vi "AMZ_S3_APIHLP_Parse HEAD Object Result.vi"(8 "error in (no error)":errorcluster, 11 "Response header":string) -> (0 "error out":errorcluster, 3 "HeadObjectResult":T1)   [LabVIEW 2015, in "LV Interface for Amazon S3.lvlib"]
uses:
  LV Interface for Amazon S3.lvlib
  Typedefs/AMZ_S3_API_HEADObjectResult.ctl
  Typedefs/AMZ_S3_API_GETObjectResult.ctl
  Typedefs/AMZ_S3_Key-Value pair.ctl
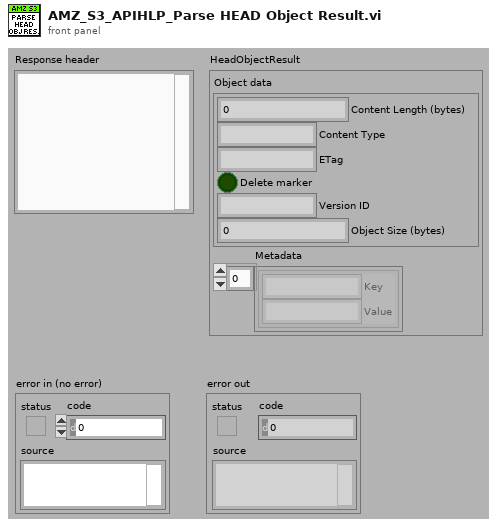
[diagram p1: front panel]
types:
  T1 = typedef "LV Interface for Amazon S3.lvlib/AMZ_S3_API_HEADObjectResult.ctl" = cluster{"Object data":T2, "Metadata":T3[]}
  T2 = typedef "LV Interface for Amazon S3.lvlib/AMZ_S3_API_GETObjectResult.ctl" = cluster{"Content Length (bytes)":u64, "Content Type":string, "ETag":string, "Delete marker":bool, "Version ID":string, "Object Size (bytes)":u64}
  T3 = typedef "LV Interface for Amazon S3.lvlib/AMZ_S3_Key-Value pair.ctl" = cluster{"Key":string, "Value":string}
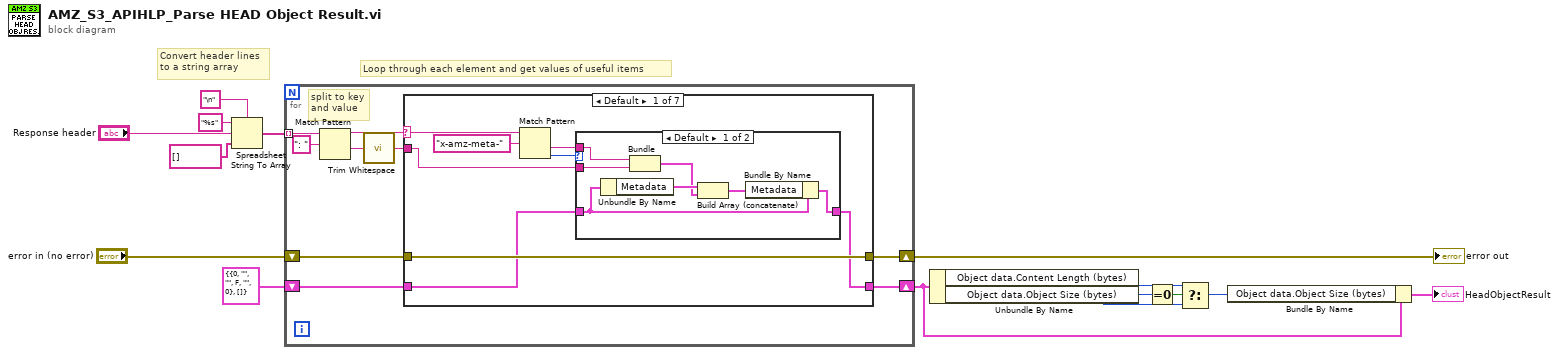
[diagram p0: block diagram]
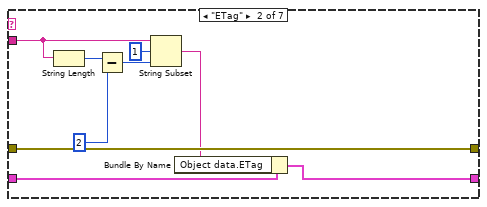
[diagram p3: hidden frame]
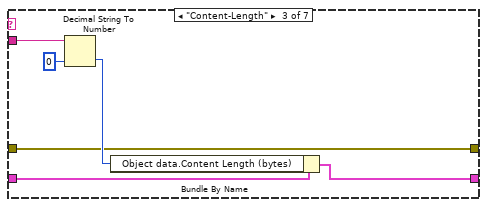
[diagram p4: hidden frame]
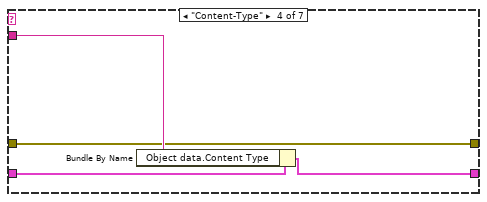
[diagram p5: hidden frame]
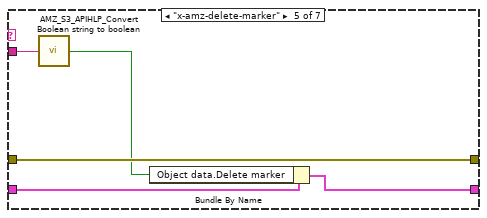
[diagram p6: hidden frame]
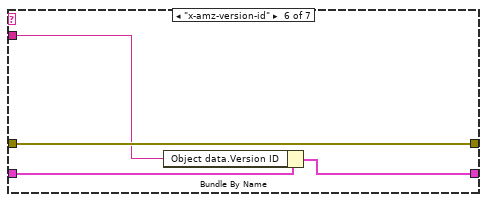
[diagram p7: hidden frame]
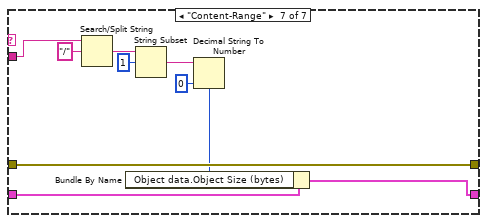
[diagram p8: hidden frame]
diagram:
  # "Loop through each element and get values of useful items"
  # "Convert header lines\nto a string array"
  n1 = Spreadsheet String To Array(delimiter (Tab)="\n", format string="%s", spreadsheet string="Response header", array type (2D Dbl)=string[] []) -> (array=w11:string[])
  n2 = for {
    tunnel: w11 -> [w23] mode=indexing
    shift-right: [w19] -> w7
    shift-left: "error in (no error)" -> [w20]
    shift-right: [w17] -> w3
    shift-left: T1 {"Object data"={"Content Length (bytes)"=0, "Content Type"="", "ETag"="", "Delete marker"=FALSE, "Version ID"="", "Object Size (bytes)"=0}, "Metadata"=[]} ("HeadObjectResult") -> [w18]
    # "split to key\nand value"
    n3 = Match Pattern(string=w23, regular expression=": ") -> (before substring=w21:string, after substring=w16:string)  [unwired: 1 in, 2 out]
    n4 = call <vilib>:"Trim Whitespace.vi"("string"=w16) -> ("trimmed string"=w15:string)  [unwired: 1 in]
    n5 = case shown="Default" w21 {
      selector: w21 -> [w30 _ _ _ _ _ _]
      tunnel: [w31 w48 w49 w55 w61 w65 w73] -> w19
      tunnel: w20 -> [w31 w48 w49 w55 w61 w65 w73]
      tunnel: w15 -> [w26 w46 w54 w57 w60 w64 w72]
      tunnel: w18 -> [w25 w42 w52 w58 w63 w67 w71]
      tunnel: [w24 w40 w50 w56 w62 w66 w70] -> w17
      frame Default {
        n6 = Match Pattern(string=w30, regular expression="x-amz-meta-") -> (after substring=w27:string, offset past match=w28:i32)  [unwired: 1 in, 2 out]
        n7 = case shown="Default" w28 {
          tunnel: w27 -> [w38 _]
          tunnel: w26 -> [w37 _]
          tunnel: w25 -> [w34 w39]
          tunnel: [w32 w39] -> w24
          frame Default {
            n8 = Unbundle By Name(w34) -> ("Metadata"=w36:T3[])
            n9 = Bundle(w38, "trimmed string"=w37) -> (w35:cluster{string, "trimmed string":string})  [unwired: 1 in]
            n10 = Build Array (concatenate)(w36, w35) -> (w33:T3[])
            n11 = Bundle By Name(cluster=w34, "Metadata"=w33) -> (w32:T1)
          }
          frame -1 {
          }
        }
      }
      frame "ETag" {
        n12 = String Length(string=w46) -> (length=w45:i32)
        n13 = Subtract(x=w45, y=2) -> (x-y=w44:i32)
        n14 = String Subset(string=w46, offset (0)=1, length (rest)=w44) -> (substring=w41:string)
        n15 = Bundle By Name(cluster=w42, "Object data.ETag"=w41) -> (w40:T1)
      }
      frame "Content-Length" {
        n16 = Decimal String To Number(string=w54, default (0L)=u64 0 ("default (0 I32)")) -> (number=w51:u64)  [unwired: 1 in, 1 out]
        n17 = Bundle By Name(cluster=w52, "Object data.Content Length (bytes)"=w51) -> (w50:T1)
      }
      frame "Content-Type" {
        n18 = Bundle By Name(cluster=w58, "Object data.Content Type"=w57) -> (w56:T1)
      }
      frame "x-amz-delete-marker" {
        n19 = call "AMZ_S3_APIHLP_Convert Boolean string to boolean.vi"("Boolean string in"=w60) -> ("Boolean out"=w59:bool)  [unwired: 4 in]
        n20 = Bundle By Name(cluster=w63, "Object data.Delete marker"=w59) -> (w62:T1)
      }
      frame "x-amz-version-id" {
        n21 = Bundle By Name(cluster=w67, "Object data.Version ID"=w64) -> (w66:T1)
      }
      frame "Content-Range" {
        n22 = Search/Split String(string=w72, search string/char (-)="/") -> (match + rest of string=w76:string)  [unwired: 1 in, 2 out]
        n23 = String Subset(string=w76, offset (0)=1) -> (substring=w74:string)  [unwired: 1 in]
        n24 = Decimal String To Number(string=w74, default (0L)=u64 0) -> (number=w69:u64)  [unwired: 1 in, 1 out]
        n25 = Bundle By Name(cluster=w71, "Object data.Object Size (bytes)"=w69) -> (w70:T1)
      }
    }
  }
  "error out" <- w7
  n26 = Unbundle By Name(w3) -> ("Object data.Content Length (bytes)"=w5:u64, "Object data.Object Size (bytes)"=w4:u64)
  n27 = Equal To 0?(x=w4) -> (x = 0?=w6:bool)
  n28 = Select(t=w5, s=w6, f=w4) -> (s? t:f=w2:u64)
  n29 = Bundle By Name(cluster=w3, "Object data.Object Size (bytes)"=w2) -> (→"HeadObjectResult":T1)
